vi "Check Folder or Create.vi"(0 "path":path, 11 "error in (no error)":errorcluster) -> (4 "dup path":path, 15 "error out":errorcluster)   [LabVIEW 2019]
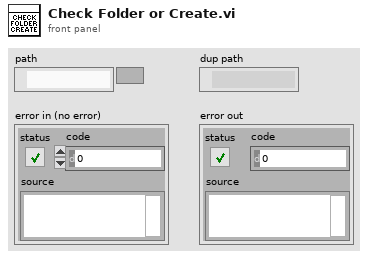
[diagram p1: front panel]
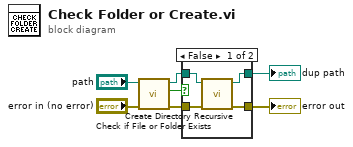
[diagram p0: block diagram]
diagram:
  n1 = call <vilib>:"Check if File or Folder Exists.vi"("error in (no error)"="error in (no error)", "path"="path") -> ("error out"=w3:errorcluster, "file or folder exists?"=w5:bool, "dup path"=w2:path)  [unwired: 7 in]
  n2 = case shown="False" w5 {
    tunnel: w2 -> [w11 w13]
    tunnel: w3 -> [w10 w12]
    tunnel: [w9 w13] -> w7
    tunnel: [w8 w12] -> w6
    frame False {
      n3 = call <vilib>:"Create Directory Recursive.vi"("error in (no error)"=w10, "directory"=w11) -> ("error out"=w8:errorcluster, "directory copy"=w9:path)  [unwired: 3 in, 1 out]
    }
    frame True {
    }
  }
  "dup path" <- w7
  "error out" <- w6
